vi "CopyPixmapToImageOuptutMaskARGB.vi"(8 "error in (no error)":errorcluster, 9 "Greyscale Image Mask":refnum<data-value>, 10 "ARGB Image Destination":refnum<data-value>, 11 "Pixmap Image Data":T1) -> (0 "error out":errorcluster, 2 "Greyscale Image Mask (duplicate)":refnum<data-value>, 3 "ARGB Image Destination (duplicate)":refnum<data-value>)   [LabVIEW 2020, in "g_ar_toolkit.image.lvlib"]
uses:
  g_ar_toolkit.image.lvlib
  <vilib>/picture/picture.llb/imagedata.ctl
  FixPixmapColourArraySize.vi
  Default8bitColourMap.vi
  <vilib>/Utility/error.llb/Error Cluster From Error Code.vi
  80b1166a-8c06-443b-b271-eb6a715622f7.vi
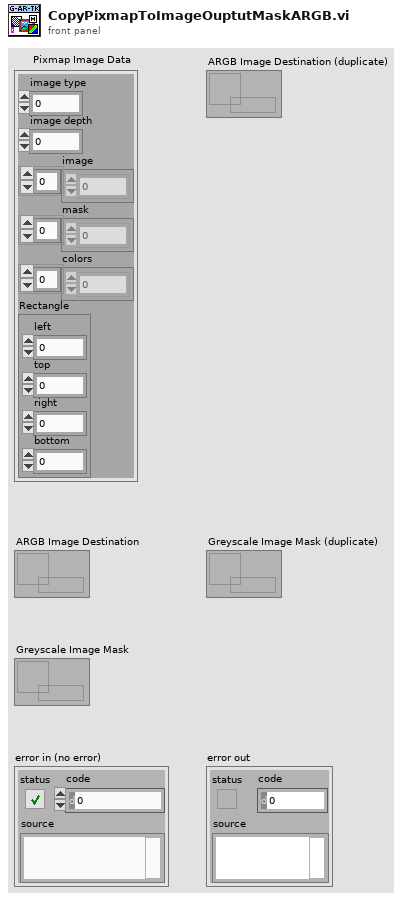
[diagram p1: front panel]
types:
  T1 = typedef "imagedata.ctl" = cluster{"image type":i32, "image depth":i32, "image":u8[], "mask":u8[], "colors":u32[], "Rectangle":cluster{"left":i16, "top":i16, "right":i16, "bottom":i16}}
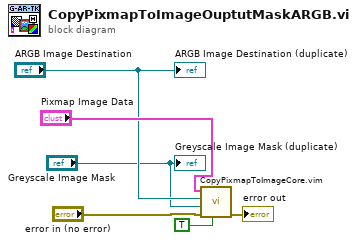
[diagram p0: block diagram]
diagram:
  n1 = call "CopyPixmapToImageCore.vim"("Has Mask"=TRUE, "error in (no error)"="error in (no error)", "Mask Image"="Greyscale Image Mask", "Destination Image"="ARGB Image Destination", "image data"="Pixmap Image Data") -> ("error out"=→"error out":errorcluster)  [unwired: 6 in]
  "ARGB Image Destination (duplicate)" <- "ARGB Image Destination"
  "Greyscale Image Mask (duplicate)" <- "Greyscale Image Mask"
